vi "build Object Information payload.vi"(8 "TransportType":T2, 9 "OrderType":T1, 10 "Time":dbl, 11 "objectInstanceHandle":u64) -> (3 "interaction_attribute_type":T3)   [LabVIEW 2019, in "HLA Custom Device Engine.lvlib"]
uses:
  HLA Custom Device Engine.lvlib
  _typedefs/object_info_received_type.ctl
  <vilib>/addons/hla/TransportationType.ctl
  <vilib>/addons/hla/OrderType.ctl
  <vilib>/addons/hla/openrti_rti1516eLv.lvlib
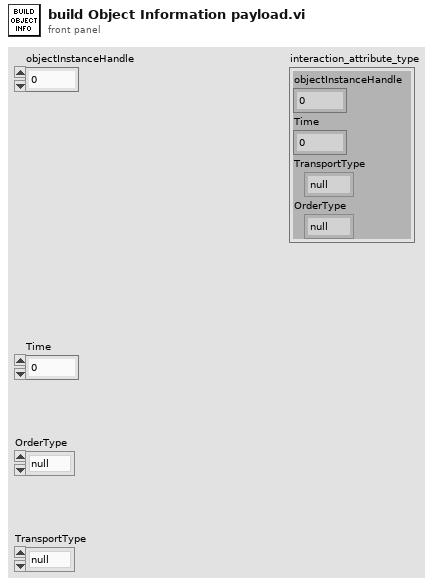
[diagram p1: front panel]
types:
  T1 = typedef "openrti_rti1516eLv.lvlib/OrderType.ctl" = enum32{"null", "RECEIVE", "TIMESTAMP"}
  T2 = typedef "openrti_rti1516eLv.lvlib/TransportationType.ctl" = enum32{"null", "RELIABLE", "BEST_EFFORT"}
  T3 = typedef "HLA Custom Device Engine.lvlib/object_info_received_type.ctl" = cluster{"objectInstanceHandle":u64, "Time":dbl, "TransportType":T2, "OrderType":T1}
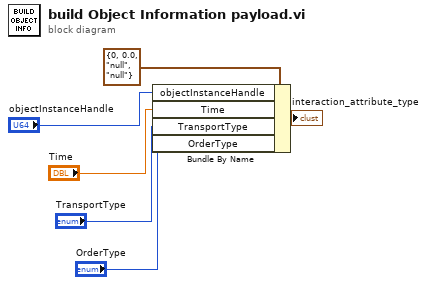
[diagram p0: block diagram]
diagram:
  n1 = Bundle By Name(cluster=T3 {"objectInstanceHandle"=0, "Time"=0.0, "TransportType"=enum."null", "OrderType"=enum."null"} ("interaction_attribute_type"), "objectInstanceHandle"="objectInstanceHandle", "Time"="Time", "TransportType"="TransportType", "OrderType"="OrderType") -> (→"interaction_attribute_type":T3)
